vi "measure_max_power_stabilisation.vi"(4 "Skip pixel?":bool, 5 "Date array":string[](array[string]), 6 "Scan settings":T1={"J-V scan"=TRUE, "J-t scan"=FALSE, "Min voltage (V)"=0.0, "Max voltage (V)"=1.4, "Step (V)"=0.01, "Measurement delay (ms)"=10.0, "1st scan FB-SC"=TRUE, "Inverted structure"=FALSE, "Stabilisation time (s)"=0.0, "Stabilisation mode"=0, "Stabilisation value (V or A) "=0.0, "Step time (s)"=1.0, "Integration time"=0, "Repeat light scans"=FALSE, "Stabilisation in the dark?"=FALSE, "J-t Min (V)"=0.0, "J-t Max (V)"=1.4, "J-t Step (V)"=0.01, "Max. power stabilisation"=FALSE, "J-t 1st scan FB-SC"=TRUE, "J-t Inverted structure"=FALSE, "Max power tracking"=FALSE, "Vmp (V)"=0.7, "Total stabilisation time (s)"=100.0, "J-t best pixel only"=0, "Max power best pixel only"=0, "Vmp from J-V scan"=FALSE, "No. of repeat scans"=2.0, "Only repeat for best pixel"=0, "Stabilisation time step (s)"=1.0, "Illumination conditions"=2, "Scan rate min (V/s)"=0.1, "Scan rate max (V/s)"=1.0, "No. of scan rate steps"=1.0, "Scan rate voltage step priority"=FALSE, "Scan rate measurement delay priority"=FALSE, "J-t Illumination conditions"=0, "Max P stab. Specific voltage"=FALSE} {"J-t Illumination conditions" items=["Light only", "Dark only", "Light then dark", "Dark then light"]; "No. of scan rate steps" min=1.0 step=1.0; "Illumination conditions" items=["Light only", "Dark only", "Light then dark", "Dark then light", "Light then dark then light", "Dark then light then dark"]; "Only repeat for best pixel" items=["only for best pixel", "for best 2 pixels", "for best 3 pixels", "for best 4 pixels", "for best 5 pixels", "for best 6 pixels", "for best 7 pixels", "for all pixels"]; "No. of repeat scans" min=1.0 step=1.0; "Max power best pixel only" items=["only the best pixel", "the best 2 pixels", "the best 3 pixels", "the best 4 pixels", "the best 5 pixels", "the best 6 pixels", "the best 7 pixels", "all pixels"]; "J-t best pixel only" items=["only the best pixel", "the best 2 pixels", "the best 3 pixels", "the best 4 pixels", "the best 5 pixels", "the best 6 pixels", "the best 7 pixels", "all pixels"]; "Integration time" items=["Fast", "Normal", "High Accuracy"]; "Stabilisation mode" items=["V", "I"]; "Measurement delay (ms)" min=10.0}, 7 "Cell details cluster":T3={"Cell Position"=16, "Cell Label"="", "Pixel to measure"=0, "Area (cm^2)"=0.126, "Variable"="", "Variable value"="", "Scan settings in queue"=0, "Light or dark"="", "Measurement Type"=""} {"Pixel to measure" items=["All", "1", "2", "3", "4", "5", "6", "7", "8"]}, 8 "Intensity (no. of suns)":string, 9 "File path of JV log":path, 10 "Experiment Title":string, 11 "User Name":string) -> (3 "Jt Curve":cluster{"Y":dbl[], "Y":dbl[]}[](graph) caption="JV Curve")   [LabVIEW 2016]
uses:
  TypeDefs/scan_settings.ctl
  TypeDefs/Settings Boolean.ctl
  <vilib>/Utility/file.llb/Read Delimited Spreadsheet (DBL).vi
  C:/Program Files (x86)/National Instruments/LabVIEW 2016/instr.lib/keithley_24xx/Keithley 24XX/Keithley 24XX.lvlib
panel:
  out "File path for Jt image":path
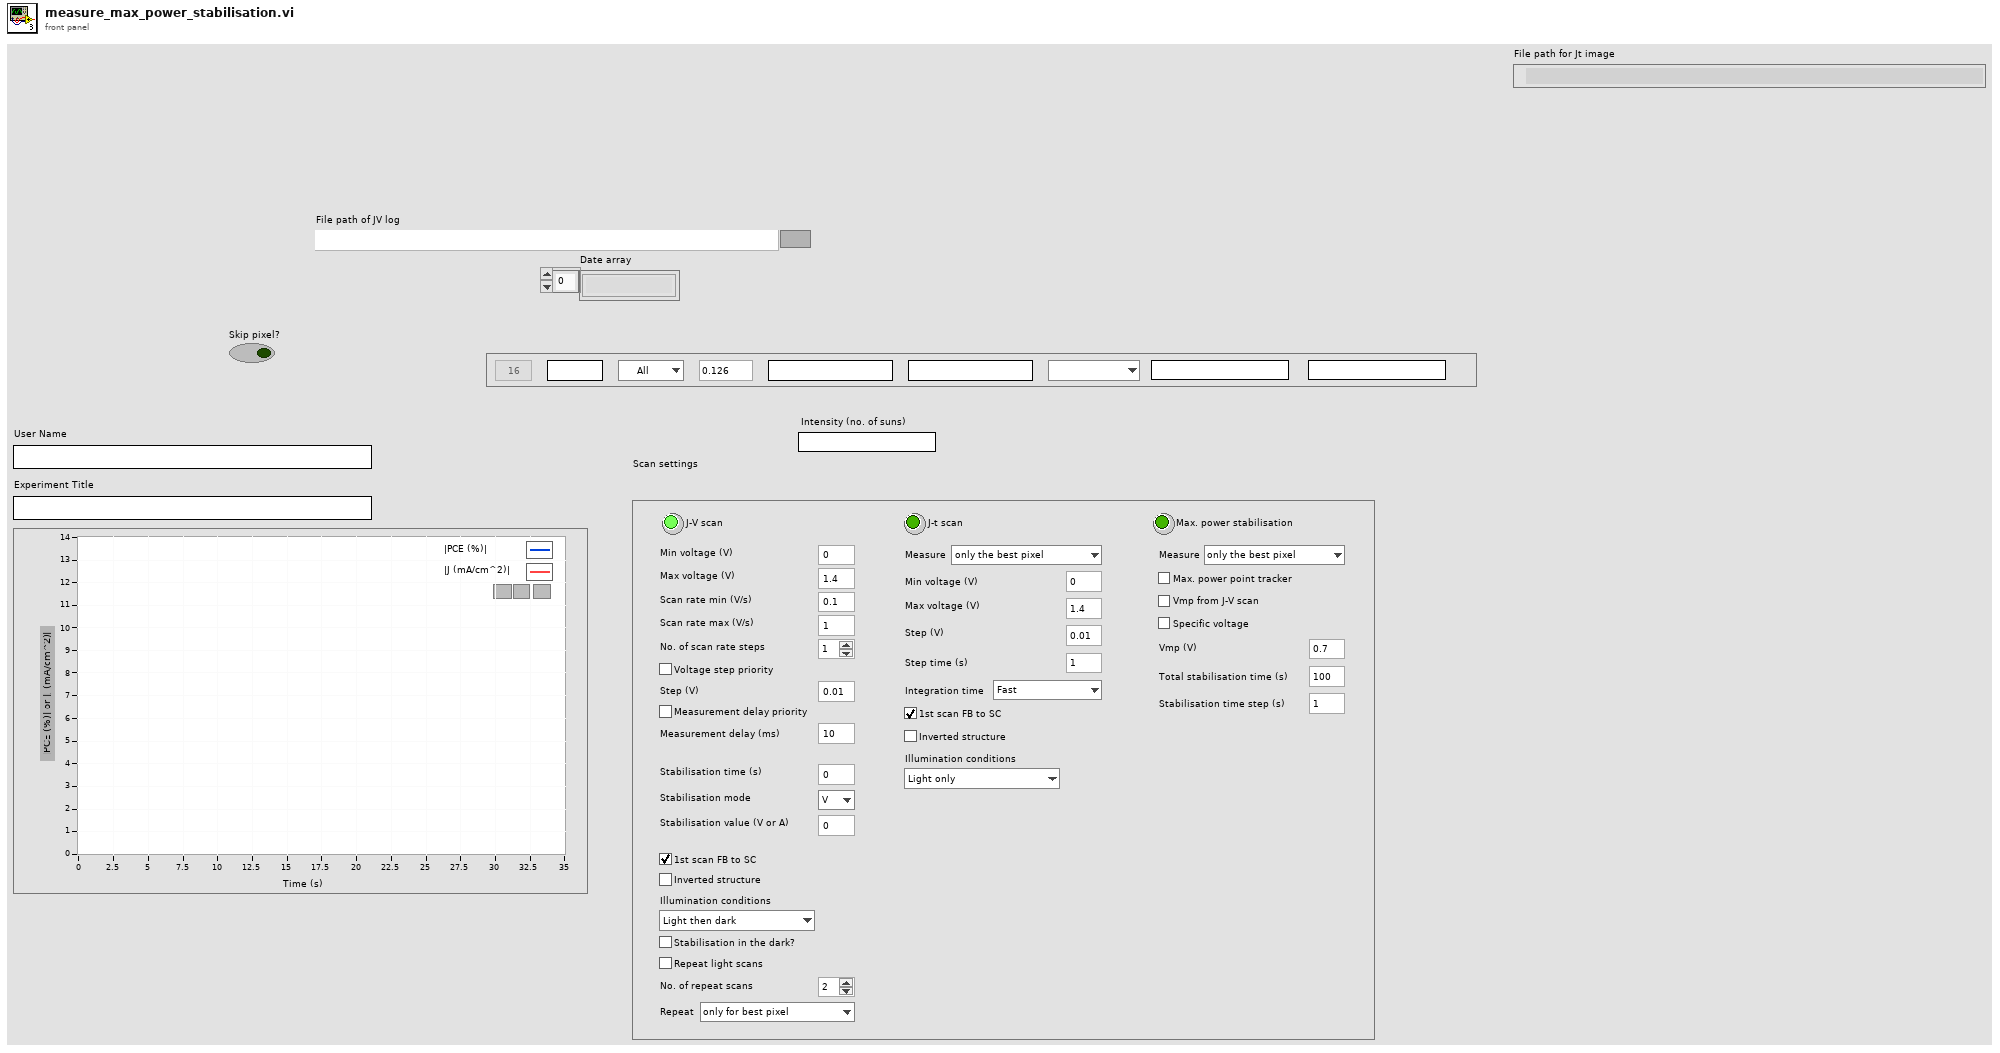
[diagram p1: front panel]
types:
  T1 = typedef "scan_settings.ctl" = cluster{"J-V scan":T2, "J-t scan":bool, "Min voltage (V)":dbl, "Max voltage (V)":dbl, "Step (V)":dbl, "Measurement delay (ms)":dbl, "1st scan FB-SC":bool, "Inverted structure":bool, "Stabilisation time (s)":dbl, "Stabilisation mode":u16, "Stabilisation value (V or A) ":dbl, "Step time (s)":dbl, "Integration time":u16, "Repeat light scans":bool, "Stabilisation in the dark?":bool, "J-t Min (V)":dbl, "J-t Max (V)":dbl, "J-t Step (V)":dbl, "Max. power stabilisation":bool, "J-t 1st scan FB-SC":bool, "J-t Inverted structure":bool, "Max power tracking":bool, "Vmp (V)":dbl, "Total stabilisation time (s)":dbl, "J-t best pixel only":u16, "Max power best pixel only":u16, "Vmp from J-V scan":bool, "No. of repeat scans":dbl, "Only repeat for best pixel":u16, "Stabilisation time step (s)":dbl, "Illumination conditions":u16, "Scan rate min (V/s)":dbl, "Scan rate max (V/s)":dbl, "No. of scan rate steps":dbl, "Scan rate voltage step priority":bool, "Scan rate measurement delay priority":bool, "J-t Illumination conditions":u16, "Max P stab. Specific voltage":bool}
  T2 = typedef "Settings Boolean.ctl" = bool
  T3 = cluster{"Cell Position":i32, "Cell Label":string, "Pixel to measure":u16, "Area (cm^2)":dbl, "Variable":string, "Variable value":string, "Scan settings in queue":u16, "Light or dark":string, "Measurement Type":string}
  T4 = typedef "imagedata.ctl" = cluster{"image type":i32, "image depth":i32, "image":u8[], "mask":u8[], "colors":u32[], "Rectangle":cluster{"left":i16, "top":i16, "right":i16, "bottom":i16}}
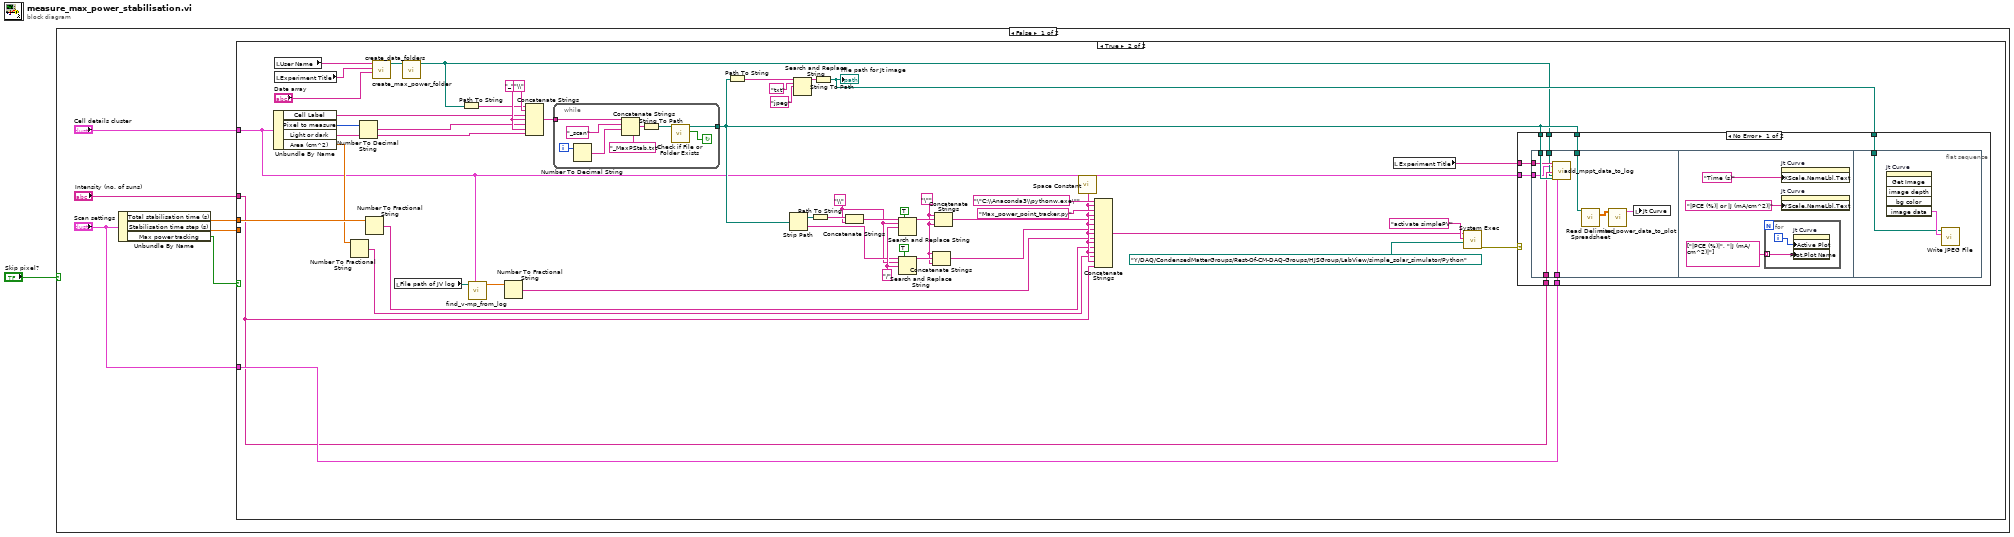
[diagram p0: block diagram]
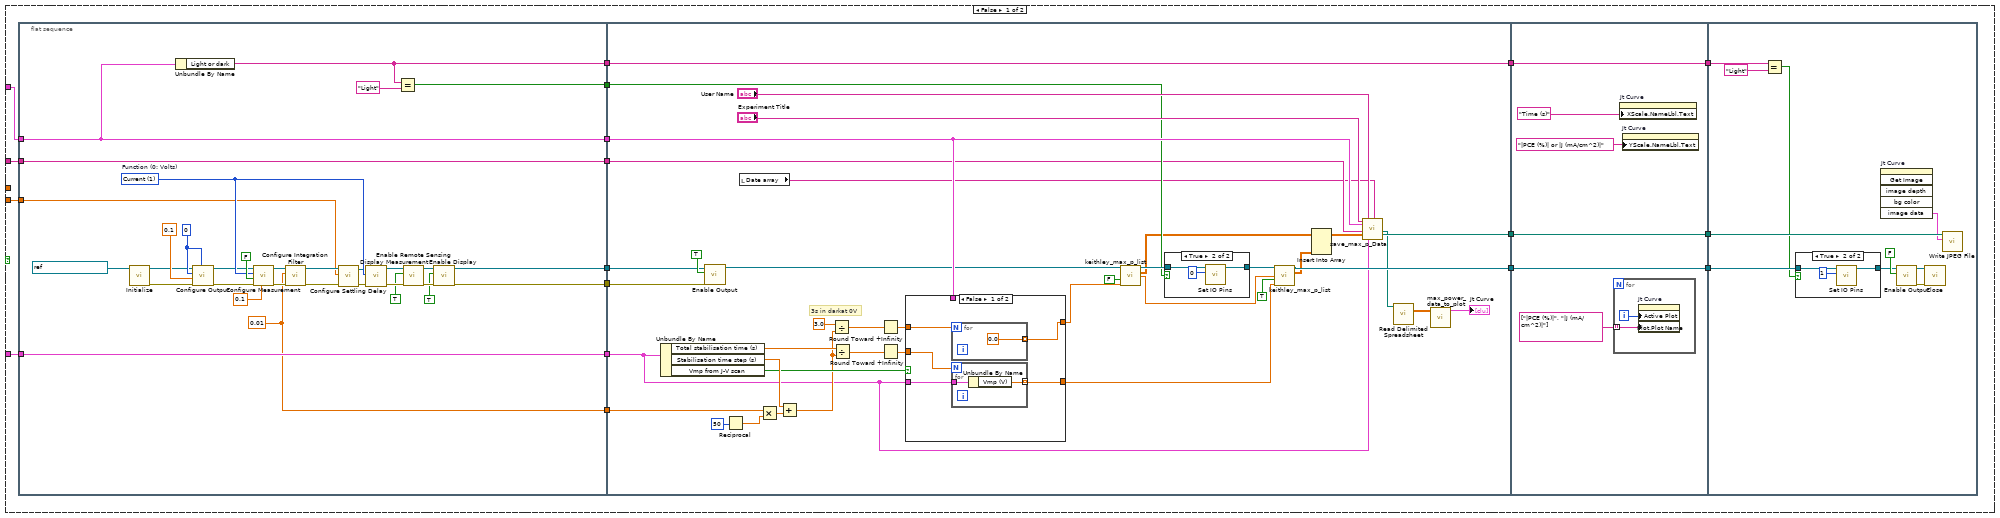
[diagram p2: hidden frame]
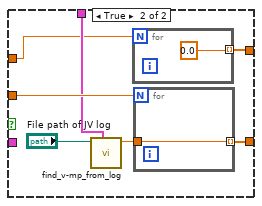
[diagram p4: hidden frame]
diagram:
  n1 = case shown="False" "Skip pixel?" {
    frame False {
      n2 = Unbundle By Name("Scan settings") -> ("Total stabilisation time (s)"=w3:dbl, "Stabilisation time step (s)"=w7:dbl, "Max power tracking"=w4:bool)
      n3 = case shown="True" w4 {
        tunnel: w7 -> [w18 _]
        tunnel: "Cell details cluster" -> [w17 w154]
        tunnel: "Scan settings" -> [w16 w158]
        tunnel: w3 -> [_ w168]
        tunnel: "Intensity (no. of suns)" -> [w14 w142]
        frame False {
          n4 = flat-sequence {
            tunnel: [w35] -> w24
            tunnel: [w36] -> w25
            tunnel: [w37] -> w23
            tunnel: w18 -> [w38]
            tunnel: [w40] -> w22
            tunnel: w17 -> [w40]
            tunnel: [w42] -> w21
            tunnel: w16 -> [w42]
            tunnel: [w39] -> w20
            tunnel: [w34] -> w19
            tunnel: [w26] -> w15
            tunnel: w14 -> [w26]
            tunnel: [w95] -> w13
            tunnel: [w97] -> w11
            tunnel: w25 -> [w64]
            tunnel: w24 -> [w63]
            tunnel: w23 -> [w88]
            tunnel: w22 -> [w81]
            tunnel: w21 -> [w58]
            tunnel: [w91] -> w9
            tunnel: w20 -> [w91]
            tunnel: w19 -> [w68]
            tunnel: w15 -> [w62]
            tunnel: w13 -> [w124]
            tunnel: [w124] -> w12
            tunnel: w11 -> [w123]
            tunnel: [w123] -> w10
            tunnel: w9 -> [w122]
            tunnel: [w122] -> w8
            tunnel: w12 -> [w130]
            tunnel: w10 -> [w133]
            tunnel: w8 -> [w127]
            frame #0 {
              w32 = 0
              w37 = 0.01
              w48 = u16 1 items=["Volts", "Current", "Resistance"]  # Function (0: Volts)
              n5 = call "Initialize.vi"("VISA resource name"=refnum<visa-resource-name> "GPIB0::24::INSTR") -> ("error out"=w27:errorcluster, "VISA resource name out"=w30:refnum<visa-resource-name>)  [unwired: 4 in, 5 out]
              n6 = Unbundle By Name(w40) -> ("Light or dark"=w39:string)
              n7 = call "Configure Output.vi"("Source Mode  (0: Voltage)"=w32, "error in (no error)"=w27, "Compliance  Level (0.1)"=0.1, "Output Level (0)"=w32, "VISA resource name"=w30) -> ("error out"=w28:errorcluster, "VISA resource name out"=w29:refnum<visa-resource-name>)  [unwired: 5 in]
              n8 = call "Configure Measurement.vi"("Manual Range (1.0)"=0.1, "error in (no error)"=w28, "Enable Auto Range (T:Enable)"=FALSE, "Function (0: Volts)"=w48, "VISA resource name"=w29) -> ("error out"=w53:errorcluster, "VISA resource name out"=w52:refnum<visa-resource-name>)  [unwired: 5 in]
              n9 = call "Configure Integration Filter.vi"("error in (no error)"=w53, "Measurement Speed (1 PLC)"=w37, "VISA resource name"=w52) -> ("error out"=w43:errorcluster, "VISA resource name out"=w46:refnum<visa-resource-name>)  [unwired: 7 in]
              n10 = call "Configure Settling Delay.vi"("error in (no error)"=w43, "Manual Settling Delay (0 sec)"=w38, "VISA resource name"=w46) -> ("error out"=w44:errorcluster, "VISA resource name out"=w45:refnum<visa-resource-name>)  [unwired: 7 in]
              n11 = call "Display Measurement.vi"("error in (no error)"=w44, "Displayed Measurement (0: Voltage)"=w48, "VISA resource name"=w45) -> ("error out"=w55:errorcluster, "VISA resource name out"=w54:refnum<visa-resource-name>)  [unwired: 7 in]
              n12 = Equal?(x=w39, y="Light") -> (x = y?=w34:bool)
              n13 = call "Enable Remote Sensing.vi"("error in (no error)"=w55, "Enable Remote Sensing (T: Enable)"=TRUE ("Enable Output (T: Enable)"), "VISA resource name"=w54) -> ("error out"=w50:errorcluster, "VISA resource name out"=w51:refnum<visa-resource-name>)  [unwired: 7 in]
              n14 = call "Enable Display.vi"("error in (no error)"=w50, "Enable Display (T: Enable)"=TRUE ("Enable Output (T: Enable)"), "VISA resource name"=w51) -> ("error out"=w35:errorcluster, "VISA resource name out"=w36:refnum<visa-resource-name>)  [unwired: 7 in]
            }
            frame #1 {
              # "3s in darkat 0V"
              n15 = Unbundle By Name(w58) -> ("Total stabilisation time (s)"=w85:dbl, "Stabilisation time step (s)"=w86:dbl, "Vmp from J-V scan"=w82:bool)
              n16 = call "Enable Output.vi"("error in (no error)"=w63, "Enable Output (T: Enable)"=TRUE ("Output (Off)"), "VISA resource name"=w64) -> ("VISA resource name out"=w73:refnum<visa-resource-name>)  [unwired: 7 in, 1 out]
              n17 = Reciprocal(x=50) -> (1/x=w90:dbl)
              n18 = local read "Date array"() -> (w59:string[])
              n19 = Multiply(x=w88, y=w90) -> (x*y=w87:dbl)
              n20 = Add(x=w86, y=w87) -> (x+y=w80:dbl)
              n21 = Divide(x=3.0, y=w80) -> (x/y=w77:dbl)
              n22 = Divide(x=w85, y=w80) -> (x/y=w78:dbl)
              n23 = Round Toward +Infinity(x=w77) -> (ceil(x): smallest int >= x=w76:dbl)
              n24 = Round Toward +Infinity(x=w78) -> (ceil(x): smallest int >= x=w84:dbl)
              n25 = case shown="False" w82 {
                tunnel: w84 -> [w106 w115]
                tunnel: w58 -> [w104 _]
                tunnel: [w105 w114] -> w83
                tunnel: w81 -> [_ w113]
                tunnel: w76 -> [w103 w112]
                tunnel: [w102 w111] -> w74
                frame False {
                  n26 = for {
                    N: w103 -> [_]
                    tunnel: [0.0 ("Vmp")] -> w102 mode=indexing
                  }
                  n27 = for {
                    N: w106 -> [_]
                    tunnel: w104 -> [w109]
                    tunnel: [w108] -> w105 mode=indexing
                    n28 = Unbundle By Name(w109) -> ("Vmp (V)"=w108:dbl)
                  }
                }
                frame True {
                  n29 = call "find_v-mp_from_log.vi"("Cell details cluster in"=w113, "File path of JV log"="File path of JV log") -> ("Vmp"=w110:dbl)  [unwired: 9 in]
                  n30 = for {
                    N: w112 -> [_]
                    tunnel: [0.0 ("Vmp")] -> w111 mode=indexing
                  }
                  n31 = for {
                    N: w115 -> [_]
                    tunnel: [w118] -> w114 mode=indexing
                    tunnel: w110 -> [w118]
                  }
                }
              }
              n32 = call "keithley_max_p_list.vi"("VISA resource name in"=w73, "Light?"=FALSE, "Voltage List"=w74) -> ("VISA resource name out"=w70:refnum<visa-resource-name>, "Data Array"=w67:dbl[][], "timestamp"=w69:sgl)  [unwired: 9 in, 1 out]
              n33 = case shown="True" w68 {
                tunnel: w70 -> [w98 w100]
                tunnel: [w98 w99] -> w75
                frame False {
                }
                frame True {
                  n34 = call "Set IO Pins.vi"("Output Pattern (0)"=0, "VISA resource name"=w100) -> ("VISA resource name out"=w99:refnum<visa-resource-name>)  [unwired: 8 in, 1 out]
                }
              }
              n35 = call "keithley_max_p_list.vi"("VISA resource name in"=w75, "t=0 timestamp"=w69, "Light?"=TRUE, "Voltage List"=w83) -> ("VISA resource name out"=w95:refnum<visa-resource-name>, "Data Array"=w66:dbl[][])  [unwired: 8 in, 2 out]
              n36 = Insert Into Array(array=w67, new element=w66) -> (w65:dbl[][])  [unwired: 2 in]
              n37 = call "save_max_p_Data.vi"("Experiment Indicator"="Experiment Title", "Cell details cluster"=w81, "Intensity (no. of suns)"=w62, "Data Array"=w65, "Username"="User Name", "Scan settings"=w58, "Date array"=w59) -> ("File path for Jt data"=w61:path, "File path for Jt image"=w97:path)  [unwired: 9 in, 2 out]
              n38 = call-poly <vilib>:"Read Delimited Spreadsheet.vi"("file path (dialog if empty)"=w61) -> ("all rows"=w60:dbl[][])  [unwired: 9 in, 5 out]
              n39 = call "max_power_data_to_plot.vi"("Data Array"=w60) -> ("JV Curve"=→"Jt Curve":cluster{"Y":dbl[], "Y":dbl[]}[])  [unwired: 10 in]
            }
            frame #2 {
              n40 = for {
                tunnel: string[] ["|PCE (%)|", "|J (mA/cm^2)|"] ("Measurement queue") -> [w125] mode=indexing
                i -> [w126]
                n41 = property on="Jt Curve" class="XYGraph (strict)"("Active Plot"=w126, "Plot.Plot Name"=w125) -> ()  [unwired: 2 in, 2 out]
              }
              n42 = property on="Jt Curve" class="XYGraph (strict)"("XScale.NameLbl.Text"="Time (s)" ("Y Scale.Name Label.Text")) -> ()  [unwired: 2 in, 2 out]
              n43 = property on="Jt Curve" class="XYGraph (strict)"("YScale.NameLbl.Text"="|PCE (%)| or |J (mA/cm^2)|" ("Y Scale.Name Label.Text")) -> ()  [unwired: 2 in, 2 out]
            }
            frame #3 {
              n44 = Equal?(x=w127, y="Light") -> (x = y?=w128:bool)
              n45 = case shown="True" w128 {
                tunnel: w130 -> [w137 w139]
                tunnel: [w137 w138] -> w129
                frame False {
                }
                frame True {
                  n46 = call "Set IO Pins.vi"("Output Pattern (0)"=1, "VISA resource name"=w139) -> ("VISA resource name out"=w138:refnum<visa-resource-name>)  [unwired: 8 in, 1 out]
                }
              }
              n47 = invoke on="Jt Curve" class="XYGraph (strict)" method="Get Image"() -> ("image data"=w132:T4)  [unwired: 6 in, 5 out]
              n48 = call "Enable Output.vi"("Enable Output (T: Enable)"=FALSE ("Output (Off)"), "VISA resource name"=w129) -> ("error out"=w135:errorcluster, "VISA resource name out"=w136:refnum<visa-resource-name>)  [unwired: 8 in]
              n49 = call "Close.vi"("error in (no error)"=w135, "VISA resource name"=w136) -> ()  [unwired: 9 in, 1 out]
              n50 = call <vilib>:"Write JPEG File.vi"("image data"=w132, "path to JPEG file"=w133) -> ()  [unwired: 8 in, 2 out]
            }
          }
        }
        frame True {
          w149 = "\"" ("string")
          w173 = "/" ("search string")
          w148 = "\\" ("search string")
          w183 = "_"
          n51 = Unbundle By Name(w154) -> ("Cell Label"=w179:string, "Pixel to measure"=w180:u16, "Light or dark"=w177:string, "Area (cm^2)"=w165:dbl)
          n52 = local read "User Name"() -> (w185:string)
          n53 = local read "Experiment Title"() -> (w186:string)
          n54 = Number To Fractional String(number=w165) -> (F-format string=w143:string)  [unwired: 3 in]
          n55 = Number To Decimal String(number=w180) -> (decimal integer string=w178:string)  [unwired: 1 in]
          n56 = Number To Fractional String(number=w168) -> (F-format string=w144:string)  [unwired: 3 in]
          n57 = call "create_data_folders.vi"("Date array"="Date array", "Experiment Indicator"=w186, "username"=w185) -> ("Data Output Folder"=w184:path)  [unwired: 8 in]
          n58 = local read "File path of JV log"() -> (w167:path)
          n59 = call "create_max_power_folder.vi"("Data Folder In"=w184) -> ("Data Output Folder"=w155:path)  [unwired: 10 in]
          n60 = Path To String(path=w155) -> (string=w174:string)
          n61 = call "find_v-mp_from_log.vi"("Cell details cluster in"=w154, "File path of JV log"=w167) -> ("Vmp"=w166:dbl)  [unwired: 9 in]
          n62 = Number To Fractional String(number=w166) -> (F-format string=w145:string)  [unwired: 3 in]
          n63 = Concatenate Strings(w174, "\\", w179, w183, w178, w183, w177) -> (w182:string)
          n64 = while {
            tunnel: w182 -> [w223]
            tunnel: [w215] -> w157
            i -> [w221]
            stop <- w216 continue-if-true
            n65 = Number To Decimal String(number=w221) -> (decimal integer string=w220:string)  [unwired: 1 in]
            n66 = Concatenate Strings(w223, "_scan", w220, "_MaxPStab.txt") -> (w217:string)
            n67 = String To Path(string=w217) -> (path=w218:path)
            n68 = call <vilib>:"Check if File or Folder Exists.vi"("path"=w218) -> ("file or folder exists?"=w216:bool, "dup path"=w215:path)  [unwired: 8 in, 1 out]
          }
          n69 = Path To String(path=w157) -> (string=w190:string)
          n70 = Strip Path(path=w157) -> (stripped path=w163:path, name=w164:string)
          n71 = Search and Replace String(input string=w190, search string="txt", replace string="jpeg") -> (result string=w187:string)  [unwired: 5 in, 3 out]
          n72 = Path To String(path=w163) -> (string=w161:string)
          n73 = String To Path(string=w187) -> (path=w169:path)
          "File path for Jt image" <- w169
          n74 = Concatenate Strings(w161, w148) -> (w162:string)
          n75 = Search and Replace String(replace all?=TRUE ("replace all? (F)"), input string=w164, search string=w148, replace string=w173) -> (result string=w171:string)  [unwired: 4 in, 3 out]
          n76 = Search and Replace String(replace all?=TRUE ("replace all? (F)"), input string=w162, search string=w148, replace string=w173) -> (result string=w176:string)  [unwired: 4 in, 3 out]
          n77 = Concatenate Strings(w149, w171, w149) -> (w146:string)
          n78 = Concatenate Strings(w149, w176, w149) -> (w147:string)
          n79 = call <vilib>:"Space Constant.vi"() -> ("String"=w150:string)
          n80 = Concatenate Strings("\"C:\\Anaconda3\\pythonw.exe\"" ("standard input"), w150, "Max_power_point_tracker.py" ("standard input"), w150, w147, w150, w146, w150, w145, w150, w144, w150, w143, w150, w142) -> (w141:string)
          n81 = local read "Experiment Title"() -> (w156:string)
          n82 = call <vilib>:"System Exec.vi"("working directory"=path "Y:/DAQ/CondensedMatterGroups/Rest-Of-CM-DAQ-Groups/HJSGroup/LabView/simple_solar_simulator/Python", "standard input"="activate simplePV", "command line"=w141) -> ("error out"=w170:errorcluster)  [unwired: 5 in, 3 out]
          n83 = case shown="No Error" w170 {
            tunnel: w157 -> [w198 _]
            tunnel: w169 -> [w197 _]
            tunnel: w158 -> [w196 _]
            tunnel: w157 -> [w195 _]
            tunnel: w142 -> [w194 _]
            tunnel: w156 -> [w193 _]
            tunnel: w155 -> [w192 _]
            tunnel: w154 -> [w191 _]
            frame No Error {
              n84 = flat-sequence {
                tunnel: w198 -> [w207]
                tunnel: w196 -> [w204]
                tunnel: w195 -> [w203]
                tunnel: w194 -> [w202]
                tunnel: w193 -> [w201]
                tunnel: w192 -> [w200]
                tunnel: w191 -> [w199]
                tunnel: w197 -> [w213]
                frame #0 {
                  n85 = call "add_mppt_data_to_log.vi"("Experiment Indicator"=w201, "Cell details cluster"=w199, "Intensity (no. of suns)"=w202, "mppt folder path"=w200, "mppt file path"=w203, "Scan settings"=w204) -> ()  [unwired: 12 in, 2 out]
                  n86 = call-poly <vilib>:"Read Delimited Spreadsheet.vi"("file path (dialog if empty)"=w207) -> ("all rows"=w206:dbl[][])  [unwired: 9 in, 5 out]
                  n87 = call "max_power_data_to_plot.vi"("Data Array"=w206) -> ("JV Curve"=w205:cluster{"Y":dbl[], "Y":dbl[]}[])  [unwired: 10 in]
                  n88 = local write "Jt Curve"(w205) -> ()
                }
                frame #1 {
                  n89 = for {
                    tunnel: string[] ["|PCE (%)|", "|J (mA/cm^2)|"] ("Measurement queue") -> [w211] mode=indexing
                    i -> [w212]
                    n90 = property on="Jt Curve" class="XYGraph (strict)"("Active Plot"=w212, "Plot.Plot Name"=w211) -> ()  [unwired: 2 in, 2 out]
                  }
                  n91 = property on="Jt Curve" class="XYGraph (strict)"("XScale.NameLbl.Text"="Time (s)" ("Y Scale.Name Label.Text")) -> ()  [unwired: 2 in, 2 out]
                  n92 = property on="Jt Curve" class="XYGraph (strict)"("YScale.NameLbl.Text"="|PCE (%)| or |J (mA/cm^2)|" ("Y Scale.Name Label.Text")) -> ()  [unwired: 2 in, 2 out]
                }
                frame #2 {
                  n93 = invoke on="Jt Curve" class="XYGraph (strict)" method="Get Image"() -> ("image data"=w214:T4)  [unwired: 6 in, 5 out]
                  n94 = call <vilib>:"Write JPEG File.vi"("image data"=w214, "path to JPEG file"=w213) -> ()  [unwired: 8 in, 2 out]
                }
              }
            }
            frame Error {
            }
          }
        }
      }
    }
    frame True {
    }
  }
